vi "OutSineFreqSet.vi"(0 "SR865 in":T1, 2 "Frequency":dbl caption="Frequency, Hz", 5 "error in":errorcluster) -> (14 "SR865 out":T1, 19 "error out":errorcluster)   [LabVIEW 2018]
uses:
  SR865.ctl
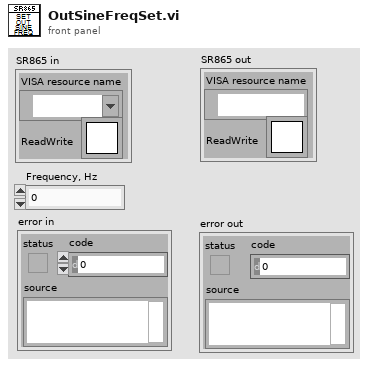
[diagram p1: front panel]
types:
  T1 = typedef "SR865.ctl" = cluster{"VISA resource name":refnum<visa-resource-name>, "ReadWrite":T2}
  T2 = typedef "Semaphore RefNum" = refnum<k1>
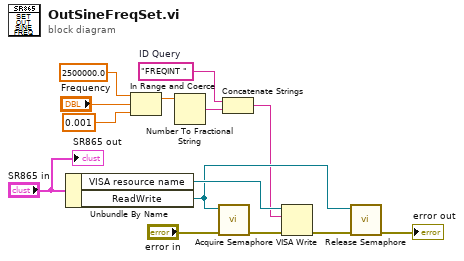
[diagram p0: block diagram]
diagram:
  w4 = "FREQINT "  # ID Query
  n1 = Unbundle By Name("SR865 in") -> ("VISA resource name"=w13:refnum<visa-resource-name>, "ReadWrite"=w9:T2)
  n2 = In Range and Coerce(upper limit=2500000.0, x="Frequency", lower limit=0.001) -> (coerced(x)=w5:dbl)  [unwired: 1 out]
  n3 = Number To Fractional String(number=w5) -> (F-format string=w3:string)  [unwired: 3 in]
  n4 = call <vilib>:"Acquire Semaphore.vi"("error in (no error)"="error in", "semaphore"=w9) -> ("error out"=w12:errorcluster)  [unwired: 3 in, 2 out]
  n5 = Concatenate Strings(w4, w3) -> (w2:string)
  n6 = VISA Write(VISA resource name=w13, write buffer=w2, error in (no error)=w12) -> (error out=w1:errorcluster)  [unwired: 2 out]
  n7 = call <vilib>:"Release Semaphore.vi"("error in (no error)"=w1, "semaphore"=w9) -> ("error out"=→"error out":errorcluster)  [unwired: 4 in, 1 out]
  "SR865 out" <- "SR865 in"
